vi "Run RT Sequence.vi"(0 "Sequence Context":T1, 1 "RT Sequence File Path":path, 2 "Gateway IP Address":string, 3 "Target (\"\": Auto-assign)":string, 4 "Sequence Timeout (s)":i32=10000, 5 "Step Timeout (ms)":dbl=10000.0, 6 "ParamNames":string[](array[string]), 7 "NumericDataType":string, 8 "ParamValues":string[](array[string]), 10 "ParamTypes":string[](array[string])) -> (14 "Report Text":string, 15 "Numeric Return Value":dbl, 16 "PassFail Return Value":bool, 17 "RT Sequence File Path out":path, 19 "error out":errorcluster)   [LabVIEW 2015, in "RTSequenceVIs.lvlib"]
uses:
  RTSequenceVIs.lvlib
  <vilib>/addons/TestStand/_TSLegacy.llb/LabVIEW Test - Sequence Context.ctl
  NationalInstruments.VeriStand.DataTypes
  <vilib>/NI Veristand/Execution/SequenceExecutionInterface/NI_VS Sequence Execution Interface.lvlib
panel:
  out "ms time elapsed (debug)":u32
  out "Timed out?":bool
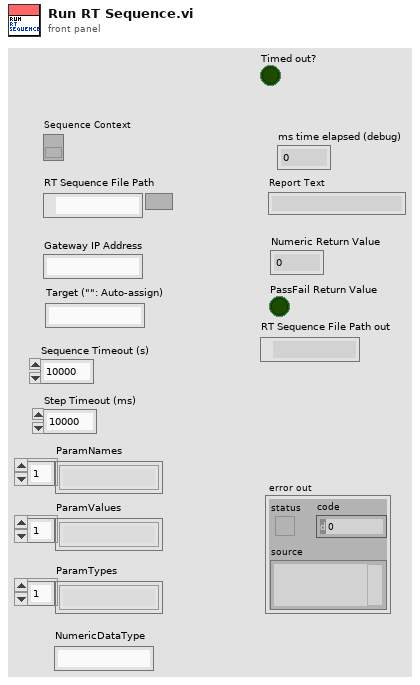
[diagram p1: front panel]
types:
  T1 = typedef "LabVIEW Test - Sequence Context.ctl" = refnum<k7>
  T2 = typedef "NI_VS Sequence Execution Interface.lvlib/Sequence Input Assignment Ref.ctl" = refnum<k24>
  T3 = typedef "NI_VS Sequence Execution Interface.lvlib/Sequence Call Ref.ctl" = refnum<k24>
  T4 = typedef "NI_VS Sequence Execution Interface.lvlib/Stimulus Profile Session Ref.ctl" = refnum<k24>
  T5 = typedef "TestStand - Status Monitor.ctl" = cluster{"Sequence Context":refnum<k7>, "Execution":refnum<k7>, "Termination Monitor":refnum<k7>}
  T6 = typedef "NI_VS Sequence Execution Interface.lvlib/Data Value Ref.ctl" = refnum<k24>
  T7 = typedef "NI_VS Sequence Execution Interface.lvlib/Deployed Session Info.ctl" = cluster{"ID":string, "Name":string, "Description":string, "Sequences":T8[], "Locked":bool}
  T8 = typedef "NI_VS Sequence Execution Interface.lvlib/Deployed Sequence Info.ctl" = cluster{"Name":string, "Path":path, "Target":string, "State":T9}
  T9 = typedef "NI_VS Sequence Execution Interface.lvlib/Sequence Execution State.ctl" = enum16{"Idle", "Running", "SingleStepping", "Paused", "Stopped"}
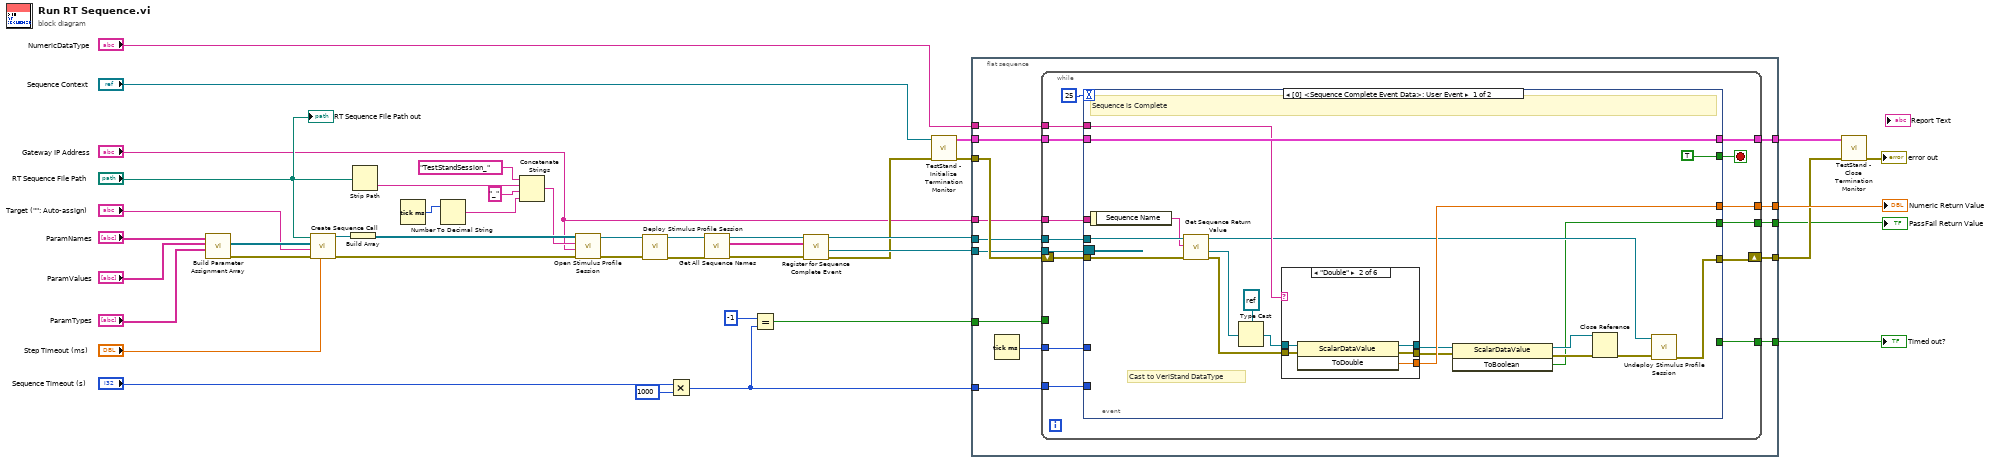
[diagram p0: block diagram]
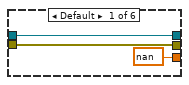
[diagram p2: hidden frame]
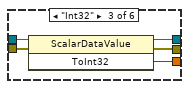
[diagram p3: hidden frame]
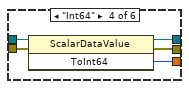
[diagram p4: hidden frame]
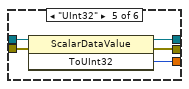
[diagram p5: hidden frame]
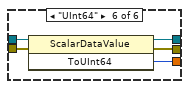
[diagram p6: hidden frame]
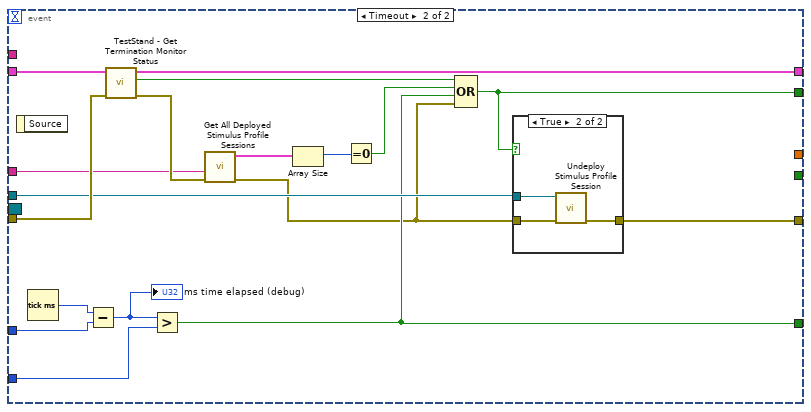
[diagram p7: hidden frame]
diagram:
  n1 = call "Build Parameter Assignment Array.vi"("ParamTypes"="ParamTypes", "ParamValues"="ParamValues", "ParamNames"="ParamNames") -> ("error out"=w40:errorcluster, "Sequence Parameter Assignment refs"=w39:T2[])  [unwired: 7 in]
  n2 = call <vilib>:"Create Sequence Call.vi"("Timeout ms (10000)"="Step Timeout (ms)", "error in (no error)"=w40, "Target (\"\": Auto-assign)"="Target (\"\": Auto-assign)", "Parameter Assignments"=w39, "Sequence File Path"="RT Sequence File Path") -> ("error out"=w7:errorcluster, "Sequence Call Ref"=w37:T3)  [unwired: 5 in]
  n3 = Build Array(w37) -> (w36:T3[])
  n4 = Strip Path(path="RT Sequence File Path") -> (name=w8:string)  [unwired: 1 out]
  n5 = Tick Count (ms)() -> (millisecond timer value=w3:u32)
  n6 = Number To Decimal String(number=w3) -> (decimal integer string=w2:string)  [unwired: 1 in]
  n7 = Concatenate Strings("TestStandSession_" ("Session Name"), w8, "_" ("string"), w2) -> (w10:string)
  n8 = call <vilib>:"Open Stimulus Profile Session.vi"("error in (no error)"=w7, "Gateway IP Address (\"\": localhost)"="Gateway IP Address", "Session Name"=w10, "Sequence Calls"=w36) -> ("error out"=w33:errorcluster, "Session Ref"=w34:T4)  [unwired: 6 in]
  n9 = call <vilib>:"Deploy Stimulus Profile Session.vi"("error in (no error)"=w33, "Session Ref in"=w34) -> ("error out"=w32:errorcluster, "Session Ref out"=w31:T4)  [unwired: 7 in, 1 out]
  n10 = Multiply(x="Sequence Timeout (s)", y=1000) -> (x*y=w23:i32)
  n11 = call <vilib>:"Get All Sequence Names.vi"("error in (no error)"=w32, "Session Ref in"=w31) -> ("error out"=w21:errorcluster, "Sequence Names out"=w19:string[], "Session Ref out"=w20:T4)  [unwired: 7 in]
  n12 = Equal?(x=-1, y=w23) -> (x = y?=w26:bool)
  n13 = call <vilib>:"Register for Sequence Complete Event.vi"("error in (no error)"=w21, "Sequence Names"=w19, "Session Ref in"=w20) -> ("error out"=w4:errorcluster, "Event Registration Refnum"=w5:refnum<event-registration>, "Session Ref out"=w18:T4)  [unwired: 4 in, 2 out]
  n14 = call <vilib>:"TestStand - Initialize Termination Monitor.vi"("error in (no error)"=w4, "Sequence Context In"="Sequence Context") -> ("error out"=w29:errorcluster, "Status Monitor Out"=w28:T5)  [unwired: 8 in]
  n15 = flat-sequence {
    tunnel: w29 -> [w57]
    tunnel: w28 -> [w56]
    tunnel: w26 -> [w55]
    tunnel: w23 -> [w54]
    tunnel: w18 -> [w53]
    tunnel: w5 -> [w52]
    tunnel: [w51] -> w14
    tunnel: [w50] -> w17
    tunnel: "NumericDataType" -> [w48]
    tunnel: [w47] -> w15
    tunnel: [w46] -> w12
    tunnel: [w45] -> w13
    tunnel: "Gateway IP Address" -> [w44]
    frame #0 {
      n16 = Tick Count (ms)() -> (millisecond timer value=w49:u32)
      n17 = while {
        tunnel: w56 -> [w66]
        tunnel: w54 -> [w63]
        tunnel: w55 -> [_]
        shift-right: [w68] -> w51
        shift-left: w57 -> [w72]
        tunnel: w53 -> [w71]
        tunnel: w52 -> [w70]
        tunnel: [w65] -> w50
        tunnel: w49 -> [w64]
        tunnel: w48 -> [w62]
        tunnel: [w61] -> w47
        tunnel: [w60] -> w46
        tunnel: [w59] -> w45
        tunnel: w44 -> [w58]
        stop <- w69 stop-if-true
        n18 = event shown="[0] <Sequence Complete Event Data>: User Event" {
          selector: w70 -> [_ _]
          dyn-events: _ -> [_ _]
          timeout: 25 -> [_ _]
          tunnel: w72 -> [w89 w136]
          tunnel: w71 -> [w88 w126]
          tunnel: [TRUE w121] -> w69
          tunnel: [w74 w122] -> w68
          tunnel: w66 -> [w90 w137]
          tunnel: [w90 w135] -> w65
          tunnel: w64 -> [_ w133]
          tunnel: w63 -> [_ w131]
          tunnel: w62 -> [w82 _]
          tunnel: [w81 _] -> w61
          tunnel: [w73 _] -> w60
          tunnel: [_ w123] -> w59
          tunnel: w58 -> [_ w129]
          event User Event {
            # "Cast to VeriStand DataType"
            # "Sequence is Complete"
            n19 = event-data() -> ("Sequence Name"=w87:string)  [unwired: 1 in]
            n20 = call <vilib>:"Get Sequence Return Value.vi"("error in (no error)"=w89, "Sequence Name"=w87, "Session Ref in"=w88) -> ("error out"=w84:errorcluster, "Data Value Ref"=w85:T6, "Session Ref out"=w75:T4)  [unwired: 5 in, 1 out]
            n21 = Type Cast(type=refnum<k24> refnum ("Node"), x=w85) -> (*(type *) &x=w83:refnum<k24>)
            n22 = case shown="\"Double\"" w82 {
              tunnel: [w92 w99 w104 w109 w114 w119] -> w80
              tunnel: [w93 w98 w103 w108 w113 w118] -> w79
              tunnel: [nan ("ToDouble") w97 w102 w107 w112 w115] -> w81
              tunnel: w83 -> [w93 w96 w100 w106 w110 w116]
              tunnel: w84 -> [w92 w95 w101 w105 w111 w117]
              frame Default {
              }
              frame "Double" {
                n23 = invoke class="ScalarDataValue" method="ToDouble"(reference=w96, error in=w95) -> (reference out=w98:refnum<k24>, error out=w99:errorcluster, "ToDouble"=w97:dbl)  [unwired: 1 in]
              }
              frame "Int32" {
                n24 = invoke class="ScalarDataValue" method="ToInt32"(reference=w100, error in=w101) -> (reference out=w103:refnum<k24>, error out=w104:errorcluster, "ToInt32"=w102:i32)  [unwired: 1 in]
              }
              frame "Int64" {
                n25 = invoke class="ScalarDataValue" method="ToInt64"(reference=w106, error in=w105) -> (reference out=w108:refnum<k24>, error out=w109:errorcluster, "ToInt64"=w107:i64)  [unwired: 1 in]
              }
              frame "UInt32" {
                n26 = invoke class="ScalarDataValue" method="ToUInt32"(reference=w110, error in=w111) -> (reference out=w113:refnum<k24>, error out=w114:errorcluster, "ToUInt32"=w112:u32)  [unwired: 1 in]
              }
              frame "UInt64" {
                n27 = invoke class="ScalarDataValue" method="ToUInt64"(reference=w116, error in=w117) -> (reference out=w118:refnum<k24>, error out=w119:errorcluster, "ToUInt64"=w115:u64)  [unwired: 1 in]
              }
            }
            n28 = invoke class="ScalarDataValue" method="ToBoolean"(reference=w79, error in=w80) -> (reference out=w77:refnum<k24>, error out=w78:errorcluster, "ToBoolean"=w73:bool)  [unwired: 1 in]
            n29 = Close Reference(reference=w77, error in (no error)=w78) -> (error out=w76:errorcluster)
            n30 = call <vilib>:"Undeploy Stimulus Profile Session.vi"("error in (no error)"=w76, "Session Ref in"=w75) -> ("error out"=w74:errorcluster)  [unwired: 8 in, 1 out]
          }
          event Timeout {
            n31 = event-data() -> ()  [unwired: 1 in, 1 out]
            n32 = Tick Count (ms)() -> (millisecond timer value=w134:u32)
            n33 = Subtract(x=w134, y=w133) -> (x-y=w132:u32)
            "ms time elapsed (debug)" <- w132
            n34 = call <vilib>:"TestStand - Get Termination Monitor Status.vi"("error in (no error)"=w136, "Status Monitor In"=w137) -> ("error out"=w130:errorcluster, "Terminating or Aborting"=w125:bool, "Status Monitor Out"=w135:T5)  [unwired: 7 in]
            n35 = Greater?(x=w132, y=w131) -> (0:w123:bool)
            n36 = call <vilib>:"Get All Deployed Stimulus Profile Sessions.vi"("error in (no error)"=w130, "Gateway IP Address (\"\": localhost)"=w129) -> ("error out"=w120:errorcluster, "Deployed Session IDs"=w128:T7[])  [unwired: 8 in]
            n37 = Array Size(array=w128) -> (size(s)=w127:i32)
            n38 = Equal To 0?(x=w127) -> (x = 0?=w124:bool)
            n39 = Compound Arithmetic op=OR(w125, w124, w123, w120) -> (w121:bool)
            n40 = case shown="True" w121 {
              tunnel: w126 -> [_ w141]
              tunnel: [w138 w140] -> w122
              tunnel: w120 -> [w138 w139]
              frame False {
              }
              frame True {
                n41 = call <vilib>:"Undeploy Stimulus Profile Session.vi"("error in (no error)"=w139, "Session Ref in"=w141) -> ("error out"=w140:errorcluster)  [unwired: 8 in, 1 out]
              }
            }
          }
        }
      }
    }
  }
  n42 = call <vilib>:"TestStand - Close Termination Monitor.vi"("error in (no error)"=w14, "Status Monitor In"=w17) -> ("error out"=→"error out":errorcluster)  [unwired: 9 in]
  "Timed out?" <- w13
  "Numeric Return Value" <- w15
  "PassFail Return Value" <- w12
  "RT Sequence File Path out" <- "RT Sequence File Path"
